vi "XIPIN_7_Series_Integrated_Block_for_PCI_Express_3_2.vi"   [LabVIEW 2017]
doc: "The Xilinx 7 Series Integrated Block for PCI Express (1-lane, 2-lane, 4-lane, and 8-lane) uses the 7-Series Integrated Hard IP Block for PCI Express in conjunction with flexible 7-Series architectural features to implement a PCI Express Base Specification v2.1 compliant PCI Express Endpoint or Root Port. Unique features of the LogiCORE Block for PCI Express are the high performance AXI Interface, optimal buffering for high bandwidth applications, and BAR checking and filtering.\n------------------------------------\n<b>Need License</b> : No\n<b>Interface</b> : AXI4-Stream"
uses:
  <vilib>/rvi/XilinxIP/XIPIN_XNode/niFpgaXIPIN.xnode
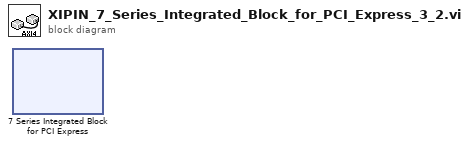
[diagram p0: block diagram]
diagram:
  n1 = xnode ("7 Series Integrated Block for PCI Express")() -> ()
